vi "LVFunction_Imop_Load_Positions_From_File.vi"(0 "path":path, 5 "dimension size":i32, 11 "error in (no error)":errorcluster) -> (4 "positions":sgl[](array[numeric]), 15 "error out":errorcluster)   [LabVIEW 2018]
doc: "Get Wavefront corrector positions from positions file.\n\n<B>file_pathIn</B> : Positions file path.\n<B>dimension size</B> : number of deformable mirror actuators\n<B>file_pathOut</B> : Positions file path.\n<B>position</B> : Positions values."
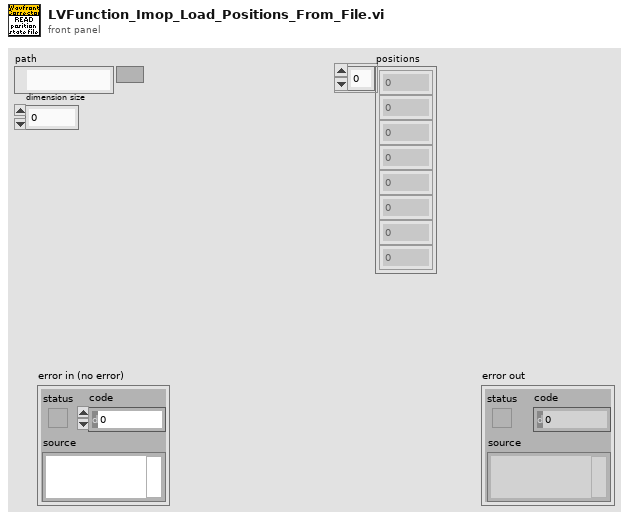
[diagram p1: front panel]
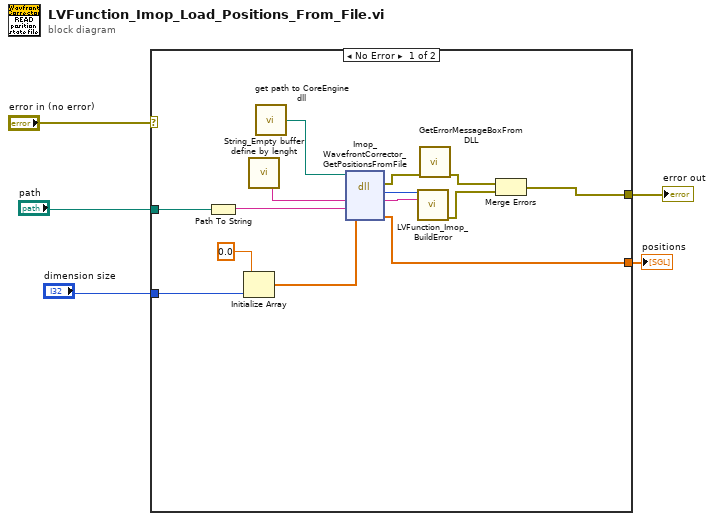
[diagram p0: block diagram]
diagram:
  n1 = case shown="No Error" "error in (no error)" {
    selector: "error in (no error)" -> [_ w20]
    tunnel: [w12 w20] -> w4
    tunnel: [w11 _] -> w3
    tunnel: "path" -> [w9 _]
    tunnel: "dimension size" -> [w6 _]
    frame No Error {
      n2 = Path To String(path=w9) -> (string=w10:string)
      n3 = Initialize Array(0.0 ("element"), w6) -> (w8:dbl[])
      n4 = call "String_Empty buffer define by lenght.vi"() -> ("Empty buffer"=w15:string)  [unwired: 1 in]
      n5 = call "get path to CoreEngine dll.vi"() -> ("path to wavekit library"=w17:path)  [unwired: 14 in, 1 out]
      n6 = dll-call lib="D:/SOFTware/CoreEngine4_Suite/SVN_trunk/LV2011_interface/DLLs/c_interface_vc100.dll" fn="Imop_WavefrontCorrector_GetPositionsFromFile"(path in=w17, "message"=w15, "pmc_file_path"=w10, "positions"=w8) -> (error out=w16:errorcluster, "return type"=w19:i32, "message"=w18:string, "positions"=w11:sgl[])  [unwired: 3 in, 1 out]
      n7 = call "LVFunction_Imop_BuildError.vi"("code"=w19, "String to Prepend to source (\"\")"=w18) -> ("error out"=w13:errorcluster)  [unwired: 13 in]
      n8 = call "GetErrorMessageBoxFromDLL.vi"("error IN"=w16) -> ("error OUT"=w14:errorcluster)  [unwired: 10 in]
      n9 = Merge Errors(w14, w13) -> (w12:errorcluster)
    }
    frame Error {
    }
  }
  "error out" <- w4
  "positions" <- w3
